vi "VFD Feedback.vi"() -> (1 "Compressor Power Output (kW)":dbl, 2 "Compressor VFD Output Frequency (Hz)":dbl, 3 "Water Pump Frequency (Hz)":dbl)   [LabVIEW 2017]
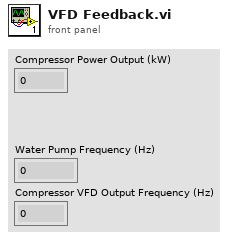
[diagram p1: front panel]
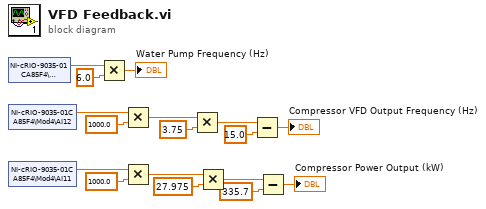
[diagram p0: block diagram]
diagram:
  n1 = shared-variable "NI-cRIO-9035-01CA85F4\\EtherCAT Master\\Device\\Mod1\\AI1"() -> (w17:dbl)  [unwired: 1 in, 1 out]
  n2 = shared-variable "NI-cRIO-9035-01CA85F4\\Mod4\\AI12"() -> (w10:dbl)  [unwired: 1 in, 1 out]
  n3 = shared-variable "NI-cRIO-9035-01CA85F4\\Mod4\\AI11"() -> (w7:dbl)  [unwired: 1 in, 1 out]
  n4 = Multiply(x=w17, y=6.0) -> (x*y=→"Water Pump Frequency (Hz)":dbl)
  n5 = Multiply(x=w10, y=1000.0) -> (x*y=w8:dbl)
  n6 = Multiply(x=w7, y=1000.0) -> (x*y=w5:dbl)
  n7 = Multiply(x=w8, y=3.75) -> (x*y=w13:dbl)
  n8 = Multiply(x=w5, y=27.975) -> (x*y=w3:dbl)
  n9 = Subtract(x=w13, y=15.0) -> (x-y=→"Compressor VFD Output Frequency (Hz)":dbl)
  n10 = Subtract(x=w3, y=335.7) -> (x-y=→"Compressor Power Output (kW)":dbl)
